vi "QUIZ1.vi"() -> ()   [LabVIEW 2020]
panel:
  in  "Pulsador":bool
  in  "Pulsador 2":bool
  in  "Pulsador 3":bool
  out "Led":bool
  out "Led 2":bool
  out "Led 3":bool
  out "Cluster 2":T1
  out "output":T2
  out "Fecha 1":T3
  out "output cluster":T2
  out "Fecha":T4
  out "Hora":T5
  out "Cluster 9":T6
  out "DELAY":dbl
  out "CONTADOR":i32
  out "Cluster 5":T7
  out "3D fix":string
  out "Cluster 4":T8
  in  "INGRESAR COMANDO":bool
  in  "COMANDOS":string
  in  "stop":bool
  out "RESPUESTA":string
  in  "TRAMA DE PRUEBA":string
  # "ESPECIFICACIONES DE LA TRAMA GGA"
  # "ESPECIFICACIONES DE LA TRAMA GSA"
  # "ESPECIFICACIONES DE LA TRAMA RMC"
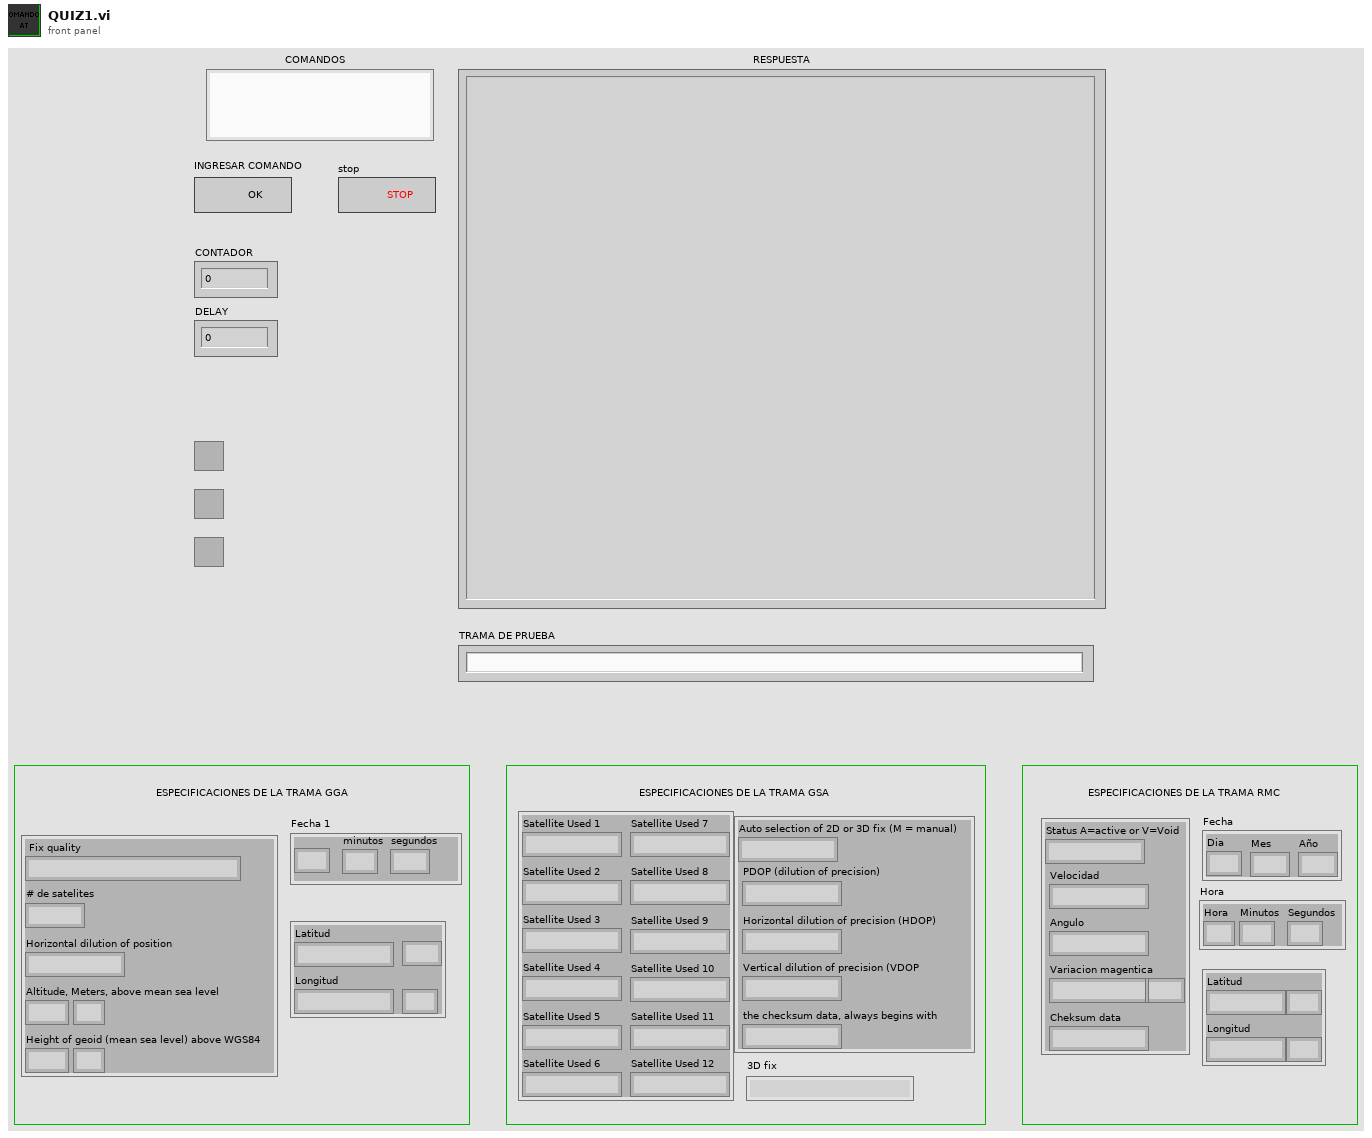
[diagram p1: front panel]
types:
  T1 = cluster{" Fix quality":string, "Horizontal dilution of position":string, "Altitude, Meters, above mean sea level":string, string, "Height of geoid (mean sea level) above WGS84":string, string, "# de satelites":string}
  T2 = cluster{"Latitud":string, string, "Longitud":string, string}
  T3 = cluster{"horas":string, "minutos":string, "segundos ":string}
  T4 = cluster{"Dia":string, "Mes":string, "Año":string}
  T5 = cluster{"Hora":string, "Segundos":string, "Minutos":string}
  T6 = cluster{"Status A=active or V=Void":string, "Velocidad":string, "Angulo":string, "Variacion magentica":string, string, "Cheksum data":string}
  T7 = cluster{"Satellite Used 1":string, "Satellite Used 2":string, "Satellite Used 3":string, "Satellite Used 4":string, "Satellite Used 5":string, "Satellite Used 6":string, "Satellite Used 7":string, "Satellite Used 8":string, "Satellite Used 9":string, "Satellite Used 10":string, "Satellite Used 11":string, "Satellite Used 12":string}
  T8 = cluster{"Auto selection of 2D or 3D fix (M = manual)":string, "PDOP (dilution of precision)":string, "Horizontal dilution of precision (HDOP)":string, "Vertical dilution of precision (VDOP":string, "the checksum data, always begins with":string}
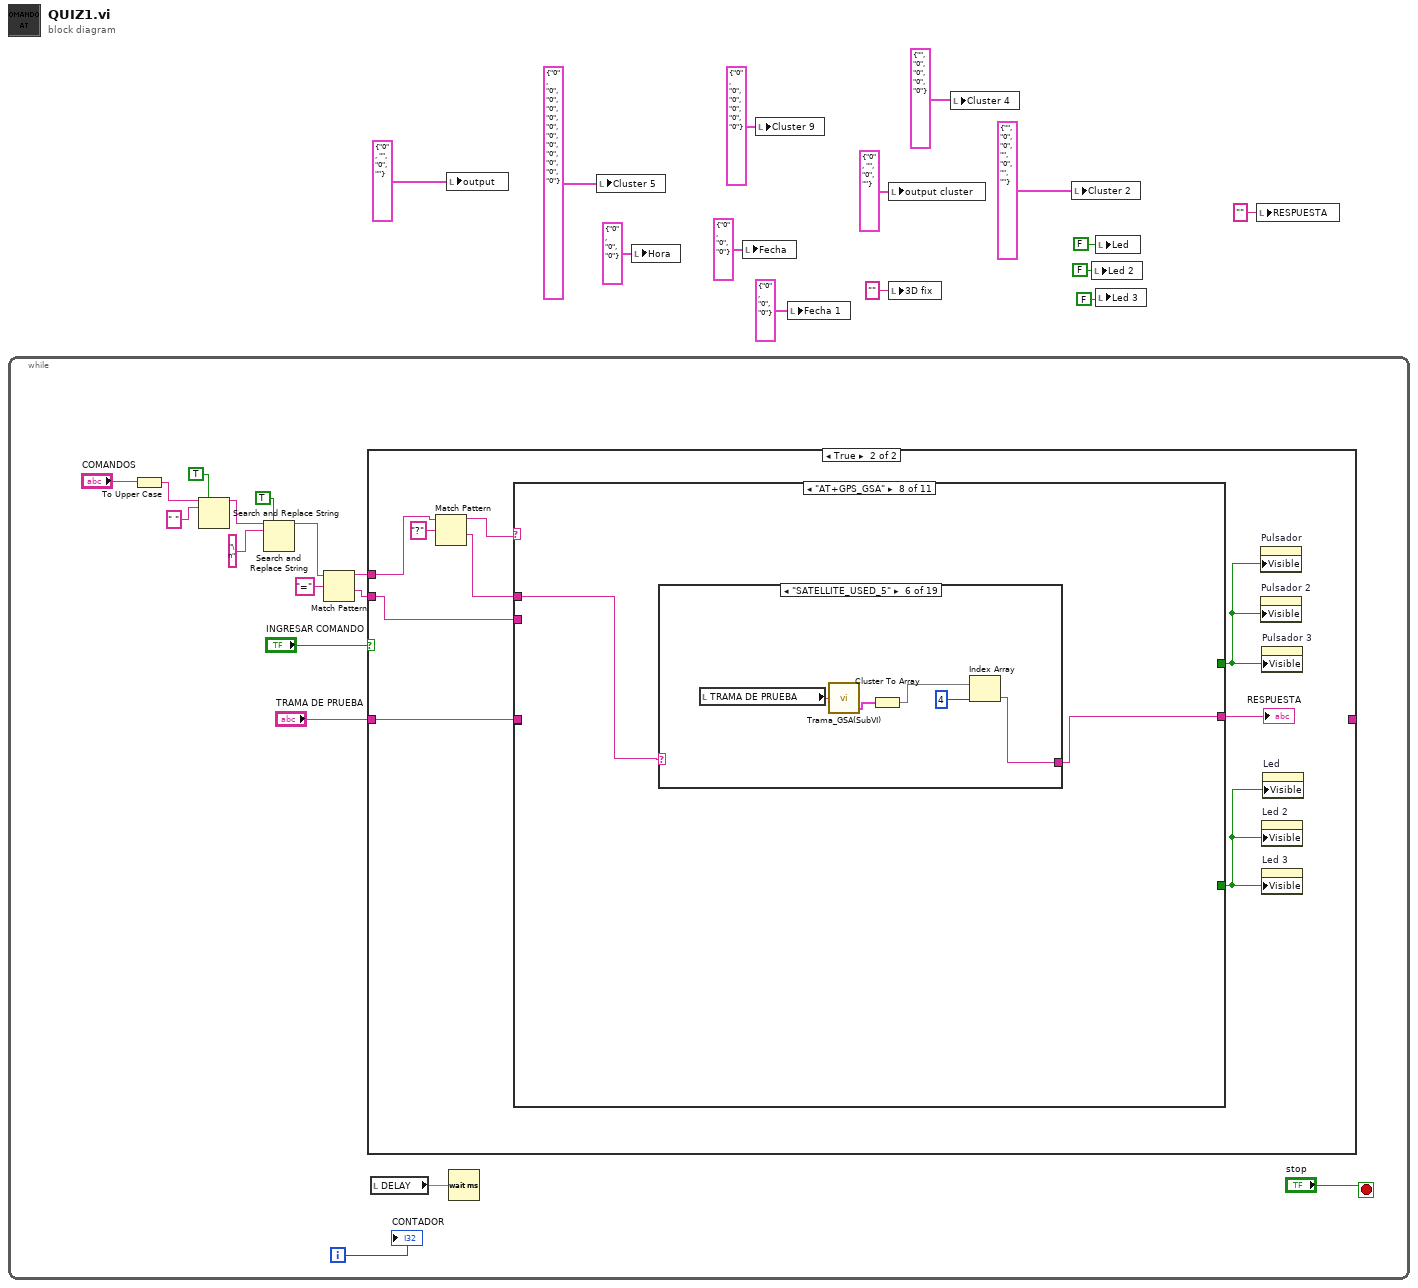
[diagram p0: block diagram]
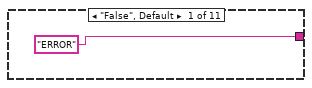
[diagram p3: hidden frame]
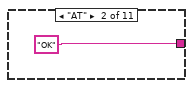
[diagram p4: hidden frame]
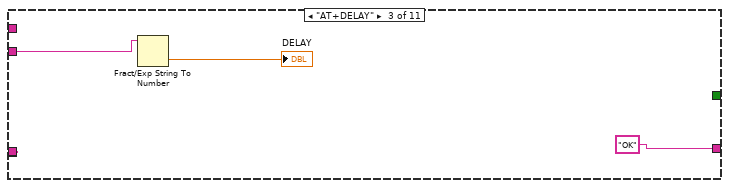
[diagram p5: hidden frame]
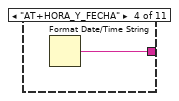
[diagram p6: hidden frame]
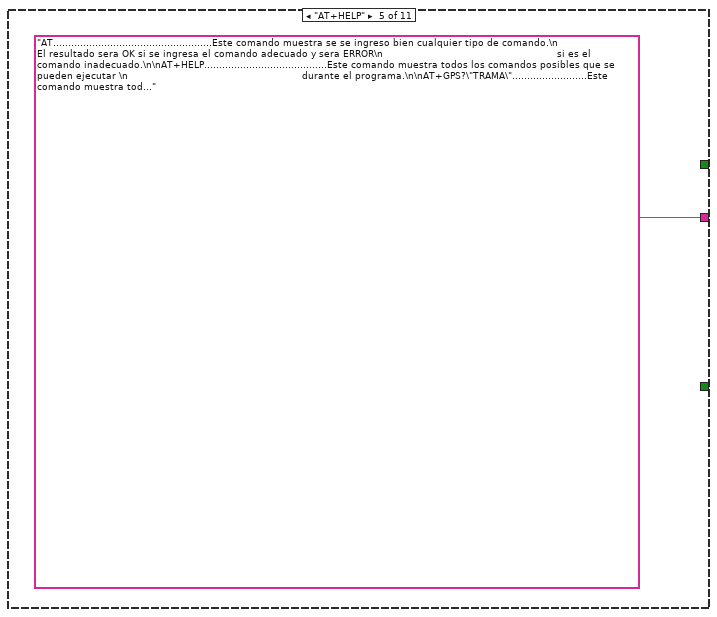
[diagram p7: hidden frame]
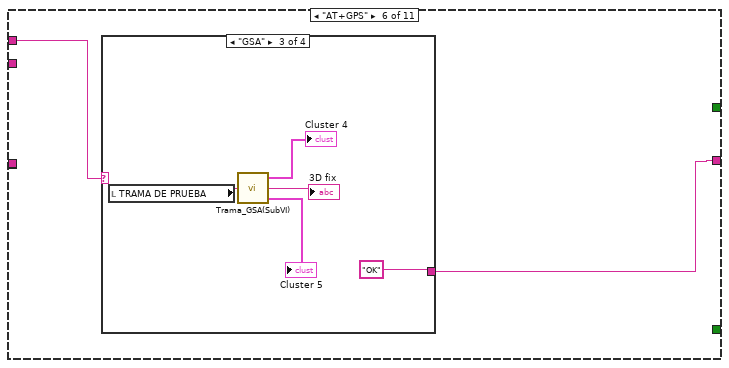
[diagram p8: hidden frame]
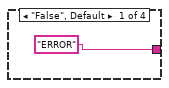
[diagram p9: hidden frame]
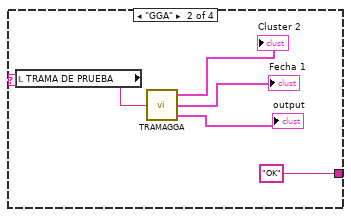
[diagram p10: hidden frame]
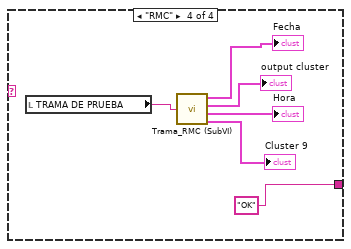
[diagram p11: hidden frame]
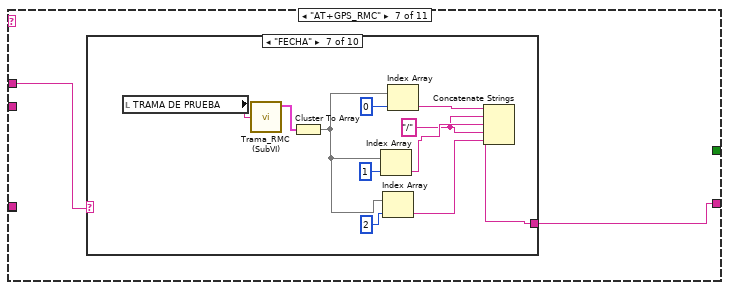
[diagram p12: hidden frame]
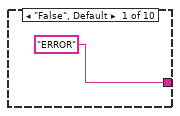
[diagram p13: hidden frame]
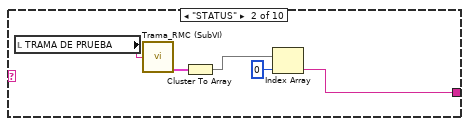
[diagram p14: hidden frame]
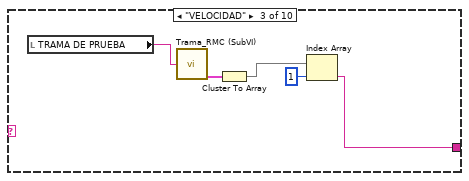
[diagram p15: hidden frame]
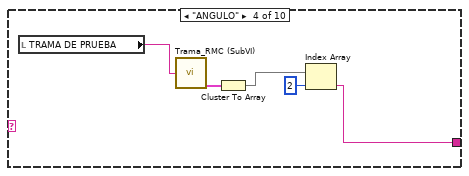
[diagram p16: hidden frame]
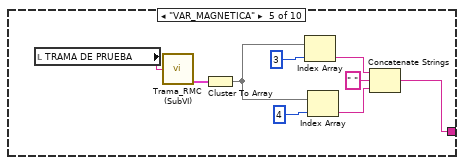
[diagram p17: hidden frame]
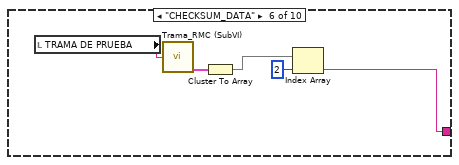
[diagram p18: hidden frame]
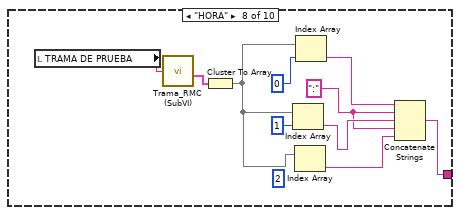
[diagram p19: hidden frame]
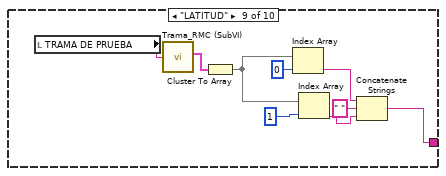
[diagram p20: hidden frame]
diagram:
  n1 = while {
    i -> [w22]
    stop <- "stop" stop-if-true
    n2 = To Upper Case(1:"COMANDOS") -> (0:w21:string)
    n3 = Search and Replace String(replace all?=TRUE ("replace all? (F)"), input string=w21, search string=" ") -> (result string=w20:string)  [unwired: 5 in, 3 out]
    n4 = Search and Replace String(replace all?=TRUE ("replace all? (F)"), input string=w20, search string="\n") -> (result string=w19:string)  [unwired: 5 in, 3 out]
    n5 = Match Pattern(string=w19, regular expression="=") -> (before substring=w25:string, after substring=w24:string)  [unwired: 1 in, 2 out]
    n6 = case shown="True" "INGRESAR COMANDO" {
      tunnel: "TRAMA DE PRUEBA" -> [w31 w34]
      tunnel: [w31 _] -> _
      tunnel: w25 -> [_ w39]
      tunnel: w24 -> [_ w36]
      frame False {
      }
      frame True {
        n7 = Match Pattern(string=w39, regular expression="?") -> (before substring=w38:string, after substring=w37:string)  [unwired: 1 in, 2 out]
        n8 = case shown="\"AT+GPS_GSA\"" w38 {
          tunnel: w37 -> [_ _ _ _ _ w50 w69 w140 w230 _ w298]
          tunnel: w36 -> [_ _ w46 _ _ _ _ _ _ _ _]
          tunnel: ["ERROR" "OK" "OK" w47 "AT.....................................................Este comando muestra se se ingreso bien cualquier tipo de comando.\n                                                          El resultado sera OK si se ingresa el comando adecuado y sera ERROR\n                                                          si es el comando inadecuado.\n\nAT+HELP.........................................Este comando muestra todos los comandos posibles que se pueden ejecutar \n                                                          durante el programa.\n\nAT+GPS?\"TRAMA\".........................Este comando muestra todos los campos de las tramas RMC,GGA O GSA.\n\nAT+GPS_RMC?\"Especificacion\"...Este comando muestra cada una de las especificaciones de la trama                          \n                                                          RMC, las cuales son:\n                                                          hora, status, latitud, longitud, velocidad, angulo, fecha, variacion\n                                                          magnetica(var_magnetica) y datos de suma de comprobacion(checksum_data). \n\nAT+GPS_GGA?\"Especificacion\"....Este comando muestra cada una de las especificaciones de la trama                          \n                                                          GGA, las cuales son:\n                                                          hora, latitud, longitud, fix quality, # de satelites que se estan rastreando(#_SAT),\n                                                          HDOP, altitud en metros(ALTIITUD), altura del geoide(ALTURA).\n                                                          \nAT+GPS_GSA?\"Especificacion\"....Este comando muestra cada una de las especificaciones de la trama                          \n                                                          GSA, las cuales son:\n                                                          Seleccion_2D_O_3D(automatica o manual), 3D_fix, Satelites_chanel_1,\n                                                          Satelites_chanel_2, Satelites_chanel_3, Satelites_chanel_4, Satelites_chanel_5,\n                                                          Satelites_chanel_6, Satelites_chanel_7, Satelites_chanel_8, Satelites_chanel_9,\n                                                          Satelites_chanel_10, Satelites_chanel_11, Satelites_chanel_12(SATELLITE_USED_n),\n                                                          PDOP, HDOP, VDOP, CHECKSUM_DATA.                                                 \n\nAT+DELAY=\"t(ms)\".......................Este comando cambia el la velocidad del contador.\n\nAT+HORA_Y_FECHA?....................Este comando muestra la hora y la fecha actual del sistema.\n\nAT+CONTADOR?...........................Este comando muestra el valor actual del contador.\n\nAT+PULSADORES?\"LED O PUL\"..Este comando muestra tres pulsadores y tres led que se pueden variar \n                                                        dependiendo de los comandos led o pulsadores. " w49 w68 w139 w229 w293 w295] -> w35
          tunnel: [_ _ w45 _ _ _ _ _ _ _ _] -> _
          tunnel: w34 -> [_ _ w45 _ _ _ _ _ _ _ _]
          tunnel: [_ _ _ _ _ _ _ _ _ _ w296] -> w33
          tunnel: [_ _ _ _ _ _ _ _ _ _ w297] -> w32
          frame "False", Default {
          }
          frame "AT" {
          }
          frame "AT+DELAY" {
            n9 = Fract/Exp String To Number(string=w46) -> (number=→"DELAY":dbl)  [unwired: 3 in, 1 out]
          }
          frame "AT+HORA_Y_FECHA" {
            n10 = Format Date/Time String() -> (date/time string=w47:string)  [unwired: 3 in]
          }
          frame "AT+HELP" {
          }
          frame "AT+GPS" {
            n11 = case shown="\"GSA\"" w50 {
              tunnel: ["ERROR" "OK" "OK" "OK"] -> w49
              frame "False", Default {
              }
              frame "GGA" {
                n12 = local read "TRAMA DE PRUEBA"() -> (w56:string)
                n13 = call "TRAMAGGA.vi"("TRAMA"=w56) -> ("Cluster 2"=→"Cluster 2":T1, "Cluster"=→"Fecha 1":T3, "output"=→"output":T2)
              }
              frame "GSA" {
                n14 = local read "TRAMA DE PRUEBA"() -> (w61:string)
                n15 = call "Trama_GSA(SubVI).vi"("TRAMA"=w61) -> ("Cluster"=→"Cluster 4":T8, "3D fix"=→"3D fix":string, "Cluster 2"=→"Cluster 5":T7)
              }
              frame "RMC" {
                n16 = local read "TRAMA DE PRUEBA"() -> (w67:string)
                n17 = call "Trama_RMC (SubVI).vi"("TRAMA"=w67) -> ("Fecha"=→"Fecha":T4, "latitud,longitud"=→"output cluster":T2, "Hora"=→"Hora":T5, "otros datos"=→"Cluster 9":T6)
              }
            }
          }
          frame "AT+GPS_RMC" {
            n18 = case shown="\"FECHA\"" w69 {
              tunnel: ["ERROR" w71 w76 w81 w88 w95 w105 w115 w125 w133] -> w68
              frame "False", Default {
              }
              frame "STATUS" {
                n19 = local read "TRAMA DE PRUEBA"() -> (w75:string)
                n20 = call "Trama_RMC (SubVI).vi"("TRAMA"=w75) -> ("otros datos"=w74:T6)  [unwired: 3 out]
                n21 = Cluster To Array(cluster=w74) -> (array=w73:string[])
                n22 = Index Array(array=w73, index=0) -> (element=w71:string)
              }
              frame "VELOCIDAD" {
                n23 = local read "TRAMA DE PRUEBA"() -> (w80:string)
                n24 = call "Trama_RMC (SubVI).vi"("TRAMA"=w80) -> ("otros datos"=w79:T6)  [unwired: 3 out]
                n25 = Cluster To Array(cluster=w79) -> (array=w78:string[])
                n26 = Index Array(array=w78, index=1) -> (element=w76:string)
              }
              frame "ANGULO" {
                n27 = local read "TRAMA DE PRUEBA"() -> (w85:string)
                n28 = call "Trama_RMC (SubVI).vi"("TRAMA"=w85) -> ("otros datos"=w84:T6)  [unwired: 3 out]
                n29 = Cluster To Array(cluster=w84) -> (array=w83:string[])
                n30 = Index Array(array=w83, index=2) -> (element=w81:string)
              }
              frame "VAR_MAGNETICA" {
                n31 = local read "TRAMA DE PRUEBA"() -> (w94:string)
                n32 = call "Trama_RMC (SubVI).vi"("TRAMA"=w94) -> ("otros datos"=w93:T6)  [unwired: 3 out]
                n33 = Cluster To Array(cluster=w93) -> (array=w90:string[])
                n34 = Index Array(array=w90, index=3) -> (element=w89:string)
                n35 = Index Array(array=w90, index=4) -> (element=w86:string)
                n36 = Concatenate Strings(w89, " " ("string"), w86) -> (w88:string)
              }
              frame "CHECKSUM_DATA" {
                n37 = local read "TRAMA DE PRUEBA"() -> (w99:string)
                n38 = call "Trama_RMC (SubVI).vi"("TRAMA"=w99) -> ("otros datos"=w98:T6)  [unwired: 3 out]
                n39 = Cluster To Array(cluster=w98) -> (array=w97:string[])
                n40 = Index Array(array=w97, index=2) -> (element=w95:string)
              }
              frame "FECHA" {
                w101 = "/" ("string")
                n41 = local read "TRAMA DE PRUEBA"() -> (w110:string)
                n42 = call "Trama_RMC (SubVI).vi"("TRAMA"=w110) -> ("Fecha"=w104:T4)  [unwired: 3 out]
                n43 = Cluster To Array(cluster=w104) -> (array=w108:string[])
                n44 = Index Array(array=w108, index=1) -> (element=w102:string)
                n45 = Index Array(array=w108, index=2) -> (element=w100:string)
                n46 = Index Array(array=w108, index=0) -> (element=w103:string)
                n47 = Concatenate Strings(w103, w101, w102, w101, w100) -> (w105:string)
              }
              frame "HORA" {
                w111 = ":" ("string")
                (unwired) 2 ("index")
                n48 = local read "TRAMA DE PRUEBA"() -> (w120:string)
                n49 = call "Trama_RMC (SubVI).vi"("TRAMA"=w120) -> ("Hora"=w114:T5)  [unwired: 3 out]
                n50 = Cluster To Array(cluster=w114) -> (array=w118:string[])
                n51 = Index Array(array=w118, index=1) -> (element=w112:string)
                n52 = Index Array(array=w118) -> (element=w113:string)  [unwired: 1 in]
                n53 = Index Array(array=w118, index=0) -> (element=w116:string)
                n54 = Concatenate Strings(w116, w111, w112, w111, w113) -> (w115:string)
              }
              frame "LATITUD" {
                n55 = local read "TRAMA DE PRUEBA"() -> (w129:string)
                n56 = call "Trama_RMC (SubVI).vi"("TRAMA"=w129) -> ("latitud,longitud"=w124:T2)  [unwired: 3 out]
                n57 = Cluster To Array(cluster=w124) -> (array=w126:string[])
                n58 = Index Array(array=w126, index=0) -> (element=w123:string)
                n59 = Index Array(array=w126, index=1) -> (element=w121:string)
                n60 = Concatenate Strings(w123, " " ("string"), w121) -> (w125:string)
              }
              frame "LONGITUD" {
                n61 = local read "TRAMA DE PRUEBA"() -> (w138:string)
                n62 = call "Trama_RMC (SubVI).vi"("TRAMA"=w138) -> ("latitud,longitud"=w132:T2)  [unwired: 3 out]
                n63 = Cluster To Array(cluster=w132) -> (array=w135:string[])
                n64 = Index Array(array=w135, index=2) -> (element=w134:string)
                n65 = Index Array(array=w135, index=3) -> (element=w130:string)
                n66 = Concatenate Strings(w134, " " ("string"), w130) -> (w133:string)
              }
            }
          }
          frame "AT+GPS_GSA" {
            n67 = case shown="\"SATELLITE_USED_5\"" w140 {
              tunnel: ["ERROR" w144 w147 w152 w157 w162 w167 w172 w177 w182 w187 w192 w197 w202 w207 w212 w217 w222 w227] -> w139
              frame "False", Default {
              }
              frame "SATELLITE_USED_1" {
                n68 = local read "TRAMA DE PRUEBA"() -> (w143:string)
                n69 = call "Trama_GSA(SubVI).vi"("TRAMA"=w143) -> ("Cluster 2"=w142:T7)  [unwired: 2 out]
                n70 = Cluster To Array(cluster=w142) -> (array=w146:string[])
                n71 = Index Array(array=w146, index=0) -> (element=w144:string)
              }
              frame "SATELLITE_USED_2" {
                n72 = local read "TRAMA DE PRUEBA"() -> (w149:string)
                n73 = call "Trama_GSA(SubVI).vi"("TRAMA"=w149) -> ("Cluster 2"=w148:T7)  [unwired: 2 out]
                n74 = Cluster To Array(cluster=w148) -> (array=w151:string[])
                n75 = Index Array(array=w151, index=1) -> (element=w147:string)
              }
              frame "SATELLITE_USED_3" {
                n76 = local read "TRAMA DE PRUEBA"() -> (w154:string)
                n77 = call "Trama_GSA(SubVI).vi"("TRAMA"=w154) -> ("Cluster 2"=w153:T7)  [unwired: 2 out]
                n78 = Cluster To Array(cluster=w153) -> (array=w156:string[])
                n79 = Index Array(array=w156, index=2) -> (element=w152:string)
              }
              frame "SATELLITE_USED_4" {
                n80 = local read "TRAMA DE PRUEBA"() -> (w160:string)
                n81 = call "Trama_GSA(SubVI).vi"("TRAMA"=w160) -> ("Cluster 2"=w159:T7)  [unwired: 2 out]
                n82 = Cluster To Array(cluster=w159) -> (array=w161:string[])
                n83 = Index Array(array=w161, index=3) -> (element=w157:string)
              }
              frame "SATELLITE_USED_5" {
                n84 = local read "TRAMA DE PRUEBA"() -> (w165:string)
                n85 = call "Trama_GSA(SubVI).vi"("TRAMA"=w165) -> ("Cluster 2"=w164:T7)  [unwired: 2 out]
                n86 = Cluster To Array(cluster=w164) -> (array=w166:string[])
                n87 = Index Array(array=w166, index=4) -> (element=w162:string)
              }
              frame "SATELLITE_USED_6" {
                n88 = local read "TRAMA DE PRUEBA"() -> (w170:string)
                n89 = call "Trama_GSA(SubVI).vi"("TRAMA"=w170) -> ("Cluster 2"=w169:T7)  [unwired: 2 out]
                n90 = Cluster To Array(cluster=w169) -> (array=w171:string[])
                n91 = Index Array(array=w171, index=5) -> (element=w167:string)
              }
              frame "SATELLITE_USED_7" {
                n92 = local read "TRAMA DE PRUEBA"() -> (w175:string)
                n93 = call "Trama_GSA(SubVI).vi"("TRAMA"=w175) -> ("Cluster 2"=w174:T7)  [unwired: 2 out]
                n94 = Cluster To Array(cluster=w174) -> (array=w176:string[])
                n95 = Index Array(array=w176, index=6) -> (element=w172:string)
              }
              frame "SATELLITE_USED_8" {
                n96 = local read "TRAMA DE PRUEBA"() -> (w180:string)
                n97 = call "Trama_GSA(SubVI).vi"("TRAMA"=w180) -> ("Cluster 2"=w179:T7)  [unwired: 2 out]
                n98 = Cluster To Array(cluster=w179) -> (array=w181:string[])
                n99 = Index Array(array=w181, index=7) -> (element=w177:string)
              }
              frame "SATELLITE_USED_9" {
                n100 = local read "TRAMA DE PRUEBA"() -> (w185:string)
                n101 = call "Trama_GSA(SubVI).vi"("TRAMA"=w185) -> ("Cluster 2"=w184:T7)  [unwired: 2 out]
                n102 = Cluster To Array(cluster=w184) -> (array=w186:string[])
                n103 = Index Array(array=w186, index=8) -> (element=w182:string)
              }
              frame "SATELLITE_USED_10" {
                n104 = local read "TRAMA DE PRUEBA"() -> (w190:string)
                n105 = call "Trama_GSA(SubVI).vi"("TRAMA"=w190) -> ("Cluster 2"=w189:T7)  [unwired: 2 out]
                n106 = Cluster To Array(cluster=w189) -> (array=w191:string[])
                n107 = Index Array(array=w191, index=9) -> (element=w187:string)
              }
              frame "SATELLITE_USED_11" {
                n108 = local read "TRAMA DE PRUEBA"() -> (w195:string)
                n109 = call "Trama_GSA(SubVI).vi"("TRAMA"=w195) -> ("Cluster 2"=w194:T7)  [unwired: 2 out]
                n110 = Cluster To Array(cluster=w194) -> (array=w196:string[])
                n111 = Index Array(array=w196, index=10) -> (element=w192:string)
              }
              frame "SATELLITE_USED_12" {
                n112 = local read "TRAMA DE PRUEBA"() -> (w200:string)
                n113 = call "Trama_GSA(SubVI).vi"("TRAMA"=w200) -> ("Cluster 2"=w199:T7)  [unwired: 2 out]
                n114 = Cluster To Array(cluster=w199) -> (array=w201:string[])
                n115 = Index Array(array=w201, index=11) -> (element=w197:string)
              }
              frame "SELECCION_2D_O_3D" {
                n116 = local read "TRAMA DE PRUEBA"() -> (w205:string)
                n117 = call "Trama_GSA(SubVI).vi"("TRAMA"=w205) -> ("Cluster"=w203:T8)  [unwired: 2 out]
                n118 = Cluster To Array(cluster=w203) -> (array=w206:string[])
                n119 = Index Array(array=w206, index=0) -> (element=w202:string)
              }
              frame "PDOP" {
                n120 = local read "TRAMA DE PRUEBA"() -> (w210:string)
                n121 = call "Trama_GSA(SubVI).vi"("TRAMA"=w210) -> ("Cluster"=w208:T8)  [unwired: 2 out]
                n122 = Cluster To Array(cluster=w208) -> (array=w211:string[])
                n123 = Index Array(array=w211, index=1) -> (element=w207:string)
              }
              frame "HDOP" {
                n124 = local read "TRAMA DE PRUEBA"() -> (w215:string)
                n125 = call "Trama_GSA(SubVI).vi"("TRAMA"=w215) -> ("Cluster"=w213:T8)  [unwired: 2 out]
                n126 = Cluster To Array(cluster=w213) -> (array=w216:string[])
                n127 = Index Array(array=w216, index=2) -> (element=w212:string)
              }
              frame "VDOP" {
                n128 = local read "TRAMA DE PRUEBA"() -> (w220:string)
                n129 = call "Trama_GSA(SubVI).vi"("TRAMA"=w220) -> ("Cluster"=w218:T8)  [unwired: 2 out]
                n130 = Cluster To Array(cluster=w218) -> (array=w221:string[])
                n131 = Index Array(array=w221, index=3) -> (element=w217:string)
              }
              frame "CHECKSUM_DATA" {
                n132 = local read "TRAMA DE PRUEBA"() -> (w225:string)
                n133 = call "Trama_GSA(SubVI).vi"("TRAMA"=w225) -> ("Cluster"=w223:T8)  [unwired: 2 out]
                n134 = Cluster To Array(cluster=w223) -> (array=w226:string[])
                n135 = Index Array(array=w226, index=4) -> (element=w222:string)
              }
              frame "3D_FIX" {
                n136 = local read "TRAMA DE PRUEBA"() -> (w228:string)
                n137 = call "Trama_GSA(SubVI).vi"("TRAMA"=w228) -> ("3D fix"=w227:string)  [unwired: 2 out]
              }
            }
          }
          frame "AT+GPS_GGA" {
            n138 = case shown="\"HORA\"" w230 {
              tunnel: ["ERROR" w232 w237 w242 w249 w258 w269 w279 w287] -> w229
              frame "False", Default {
              }
              frame "FIX_QUALITY" {
                n139 = local read "TRAMA DE PRUEBA"() -> (w236:string)
                n140 = call "TRAMAGGA.vi"("TRAMA"=w236) -> ("Cluster 2"=w235:T1)  [unwired: 2 out]
                n141 = Cluster To Array(cluster=w235) -> (array=w234:string[])
                n142 = Index Array(array=w234, index=0) -> (element=w232:string)
              }
              frame "#_SAT" {
                n143 = local read "TRAMA DE PRUEBA"() -> (w241:string)
                n144 = call "TRAMAGGA.vi"("TRAMA"=w241) -> ("Cluster 2"=w240:T1)  [unwired: 2 out]
                n145 = Cluster To Array(cluster=w240) -> (array=w239:string[])
                n146 = Index Array(array=w239, index=1) -> (element=w237:string)
              }
              frame "HDOP" {
                n147 = local read "TRAMA DE PRUEBA"() -> (w246:string)
                n148 = call "TRAMAGGA.vi"("TRAMA"=w246) -> ("Cluster 2"=w245:T1)  [unwired: 2 out]
                n149 = Cluster To Array(cluster=w245) -> (array=w244:string[])
                n150 = Index Array(array=w244, index=2) -> (element=w242:string)
              }
              frame "ALTITUD" {
                n151 = local read "TRAMA DE PRUEBA"() -> (w255:string)
                n152 = call "TRAMAGGA.vi"("TRAMA"=w255) -> ("Cluster 2"=w254:T1)  [unwired: 2 out]
                n153 = Cluster To Array(cluster=w254) -> (array=w251:string[])
                n154 = Index Array(array=w251, index=3) -> (element=w250:string)
                n155 = Index Array(array=w251, index=4) -> (element=w247:string)
                n156 = Concatenate Strings(w250, " " ("string"), w247) -> (w249:string)
              }
              frame "ALTURA" {
                n157 = local read "TRAMA DE PRUEBA"() -> (w264:string)
                n158 = call "TRAMAGGA.vi"("TRAMA"=w264) -> ("Cluster 2"=w263:T1)  [unwired: 2 out]
                n159 = Cluster To Array(cluster=w263) -> (array=w262:string[])
                n160 = Index Array(array=w262, index=5) -> (element=w261:string)
                n161 = Index Array(array=w262, index=6) -> (element=w256:string)
                n162 = Concatenate Strings(w261, " " ("string"), w256) -> (w258:string)
              }
              frame "HORA" {
                w266 = ":" ("string")
                n163 = local read "TRAMA DE PRUEBA"() -> (w275:string)
                n164 = call "TRAMAGGA.vi"("TRAMA"=w275) -> ("Cluster"=w268:T3)  [unwired: 2 out]
                n165 = Cluster To Array(cluster=w268) -> (array=w270:string[])
                n166 = Index Array(array=w270, index=0) -> (element=w274:string)
                n167 = Index Array(array=w270, index=1) -> (element=w267:string)
                n168 = Index Array(array=w270, index=2) -> (element=w265:string)
                n169 = Concatenate Strings(w274, w266, w267, w266, w265) -> (w269:string)
              }
              frame "LATITUD" {
                (unwired) 1 ("index")
                n170 = local read "TRAMA DE PRUEBA"() -> (w283:string)
                n171 = call "TRAMAGGA.vi"("TRAMA"=w283) -> ("output"=w278:T2)  [unwired: 2 out]
                n172 = Cluster To Array(cluster=w278) -> (array=w282:string[])
                n173 = Index Array(array=w282, index=0) -> (element=w281:string)
                n174 = Index Array(array=w282) -> (element=w276:string)  [unwired: 1 in]
                n175 = Concatenate Strings(w281, " " ("string"), w276) -> (w279:string)
              }
              frame "LONGITUD" {
                n176 = local read "TRAMA DE PRUEBA"() -> (w292:string)
                n177 = call "TRAMAGGA.vi"("TRAMA"=w292) -> ("output"=w286:T2)  [unwired: 2 out]
                n178 = Cluster To Array(cluster=w286) -> (array=w291:string[])
                n179 = Index Array(array=w291, index=2) -> (element=w290:string)
                n180 = Index Array(array=w291, index=3) -> (element=w284:string)
                n181 = Concatenate Strings(w290, " " ("string"), w284) -> (w287:string)
              }
            }
          }
          frame "AT+CONTADOR" {
            n182 = local read "CONTADOR"() -> (w294:i32)
            n183 = Number To Decimal String(number=w294) -> (decimal integer string=w293:string)  [unwired: 1 in]
          }
          frame "AT+PULSADORES" {
            n184 = case shown="\"LEDS\"" w298 {
              selector: w298 -> [_ w306 w313]
              tunnel: [_ w304 _] -> w297
              tunnel: [_ _ w311] -> w296
              tunnel: ["ERROR" "OK" "OK"] -> w295
              frame "False", Default {
              }
              frame "PULSADORES" {
                n185 = Equal?(x=w306, y="PULSADORES") -> (x = y?=w304:bool)
                "Led" <- "Pulsador"
                "Led 2" <- "Pulsador 2"
                "Led 3" <- "Pulsador 3"
              }
              frame "LEDS" {
                n186 = Equal?(x=w313, y="LEDS") -> (x = y?=w311:bool)
                n187 = local read "Pulsador 3"() -> (w310:bool)
                n188 = local read "Pulsador 2"() -> (w309:bool)
                n189 = local read "Pulsador"() -> (w308:bool)
                n190 = local write "Led 2"(w309) -> ()
                n191 = local write "Led 3"(w310) -> ()
                n192 = local write "Led"(w308) -> ()
              }
            }
          }
        }
        "RESPUESTA" <- w35
        n193 = property on="Pulsador" class="Bool (strict)"("Visible"=w32) -> ()  [unwired: 2 in, 2 out]
        n194 = property on="Pulsador 2" class="Bool (strict)"("Visible"=w32) -> ()  [unwired: 2 in, 2 out]
        n195 = property on="Pulsador 3" class="Bool (strict)"("Visible"=w32) -> ()  [unwired: 2 in, 2 out]
        n196 = property on="Led 2" class="Bool (strict)"("Visible"=w33) -> ()  [unwired: 2 in, 2 out]
        n197 = property on="Led 3" class="Bool (strict)"("Visible"=w33) -> ()  [unwired: 2 in, 2 out]
        n198 = property on="Led" class="Bool (strict)"("Visible"=w33) -> ()  [unwired: 2 in, 2 out]
      }
    }
    n199 = local read "DELAY"() -> (w23:dbl)
    n200 = Wait (ms)(milliseconds to wait=w23) -> ()  [unwired: 1 out]
    "CONTADOR" <- w22
  }
  n201 = local write "output"(T2 {"Latitud"="0", "", "Longitud"="0", ""} ("output")) -> ()
  n202 = local write "Cluster 5"(T7 {"Satellite Used 1"="0", "Satellite Used 2"="0", "Satellite Used 3"="0", "Satellite Used 4"="0", "Satellite Used 5"="0", "Satellite Used 6"="0", "Satellite Used 7"="0", "Satellite Used 8"="0", "Satellite Used 9"="0", "Satellite Used 10"="0", "Satellite Used 11"="0", "Satellite Used 12"="0"} ("Cluster 5")) -> ()
  n203 = local write "Hora"(T5 {"Hora"="0", "Segundos"="0", "Minutos"="0"} ("Hora")) -> ()
  n204 = local write "Fecha"(T4 {"Dia"="0", "Mes"="0", "Año"="0"} ("Fecha")) -> ()
  n205 = local write "Cluster 9"(T6 {"Status A=active or V=Void"="0", "Velocidad"="0", "Angulo"="0", "Variacion magentica"="0", "0", "Cheksum data"="0"} ("Cluster 9")) -> ()
  n206 = local write "Fecha 1"(T3 {"horas"="0", "minutos"="0", "segundos "="0"} ("Hora 1")) -> ()
  n207 = local write "output cluster"(T2 {"Latitud"="0", "", "Longitud"="0", ""} ("output cluster")) -> ()
  n208 = local write "3D fix"("" ("3D fix")) -> ()
  n209 = local write "Cluster 4"(T8 {"Auto selection of 2D or 3D fix (M = manual)"="", "PDOP (dilution of precision)"="0", "Horizontal dilution of precision (HDOP)"="0", "Vertical dilution of precision (VDOP"="0", "the checksum data, always begins with"="0"} ("Cluster 4")) -> ()
  n210 = local write "Cluster 2"(T1 {" Fix quality"="", "Horizontal dilution of position"="0", "Altitude, Meters, above mean sea level"="0", "", "Height of geoid (mean sea level) above WGS84"="0", "", "# de satelites"=""} ("Cluster 2")) -> ()
  n211 = local write "Led 2"(FALSE ("Led")) -> ()
  n212 = local write "Led"(FALSE ("Led")) -> ()
  n213 = local write "Led 3"(FALSE ("Led")) -> ()
  n214 = local write "RESPUESTA"("" ("RESPUESTA")) -> ()
